vi "PH_Beckhoff-16BB.destructor.vi"(0 "i ref in":refnum<vi>, 5 "error in(no error)":errorcluster) -> (19 "error out":errorcluster)   [LabVIEW 2014, in "PH_Beckhoff-16BB.lvlib"]
doc: "This is the destructor of a class.\n\nLicense Agreement for this software:\n\nCopyright (C)\nGesellschaft für Schwerionenforschung, GSI\nPlanckstr. 1\n64291 Darmstadt\nGermany\n\nContact: D.Beck@gsi.de \n\nThis program is free software; you can redistribute it and/or modify it under the terms of the \nGNU General Public License as published by the Free Software Foundation; either version 2 of \nthe license, or (at your option) any later version.\n\nThis program is distributed in the hope that it will be useful, but WITHOUT ANY WARRANTY; \nwithout even the implied warranty of MERCHANTABILITY or FITNESS FOR A PARTICULAR PURPOSE. See the GNU General License for more details (http://www.gnu.org).\n\nGesellschaft für Schwerionenforschung, GSI\nPlanckstr. 1, 64291 Darmstadt, Germany\nFor all questions and ideas contact: M.Richter@gsi.de, H.Brand@gsi.de or D.Beck@gsi.de.\nLast update: 16-JUN-2004"
uses:
  PH_Beckhoff-16BB.lvlib
  PH_Beckhoff/PH_Beckhoff.lvlib
  CSlibraries-extern/DimLVEvent/LVDimInterface/LVDimInterface.lvlib
  CS_Core/CSSystem/CSSystemLib/CSSystemLib.lvlib
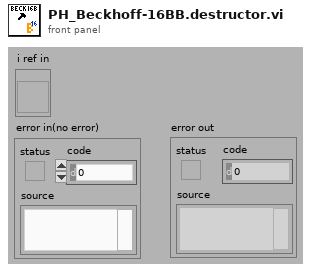
[diagram p1: front panel]
types:
  T1 = typedef "PH_Beckhoff-16BB.lvlib/PH_Beckhoff-16BB.i attribute.ctl" = cluster{"PA Chiller":cluster{"PSDB":cluster{"Status Service ID":i32, "Instance ID":i32, "Data Status":T2, "Ref Status":refnum<vi>, "Error Code":i32}, "Status":cluster{"GUI Ref":refnum<vi>, "Status Service ID":i32, "Status":T3}, "DIs":cluster{"Flow Control":cluster{"GUI Ref":refnum<vi>, "# in Data":i32}, "High-Temp":cluster{"GUI Ref":refnum<vi>, "# in Data":i32}, "Conductivity":cluster{"GUI Ref":refnum<vi>, "# in Data":i32}, "Niveau":cluster{"GUI Ref":refnum<vi>, "# in Data":i32}}, "PSDB Thread":cluster{"Ref":refnum<vi>, "Q-Ref":refnum<queue>}}, "PSDB":cluster{"Shot #":i32, "Subsystem":T4}, "Racktype":string, "PSDB Credentials":T5}
  T2 = typedef "PH_PSDBWriter.lvlib/PH_PSDBWriter.Data Status.ctl" = i16
  T3 = typedef "PH_StatusHandler.lvlib/PH_StatusHandler.Status.ctl" = i16
  T4 = typedef "PH_PSDBWriter.lvlib/PH_PSDBWriter.PHELIX-Subsystems.ctl" = i32
  T5 = typedef "PH_Common.lvlib/PH_Connection.PSDB Credentials.ctl" = cluster{"PW":string, "ID":string, "DS":string}
  T6 = enum16{"SetAttribute", "GetAttribute", "CreateAttribute", "DestroyAttribute", "DestroyAllAtributes"}
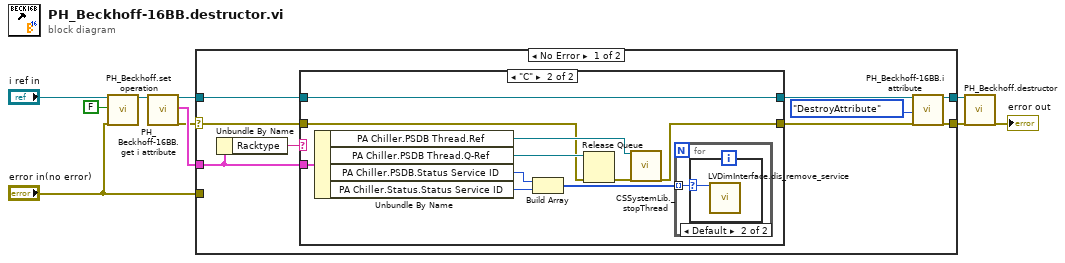
[diagram p0: block diagram]
diagram:
  n1 = call "PH_Beckhoff.set operation.vi"("VI in"="i ref in", "operation?"=FALSE, "error in (no error)"="error in(no error)") -> ("VI out"=w3:refnum<vi>)  [unwired: 15 in, 1 out]
  n2 = call "PH_Beckhoff-16BB.get i attribute.vi"("i ref in"=w3) -> ("i ref out"=w9:refnum<vi>, "i attribute"=w8:T1, "error out"=w7:errorcluster)  [unwired: 16 in]
  n3 = case shown="No Error" w7 {
    selector: w7 -> [w18 _]
    tunnel: [w14 w35] -> w6
    tunnel: [w13 w34] -> w10
    tunnel: "error in(no error)" -> [_ w34]
    tunnel: w9 -> [w19 w35]
    tunnel: w8 -> [w17 _]
    frame No Error {
      n4 = Unbundle By Name(w17) -> ("Racktype"=w16:string)
      n5 = case shown="\"C\"" w16 {
        tunnel: w19 -> [w21 w23]
        tunnel: w18 -> [w20 w24]
        tunnel: [w21 w23] -> w15
        tunnel: [w20 w22] -> w12
        tunnel: w17 -> [_ w31]
        frame Default {
        }
        frame "C" {
          n6 = Unbundle By Name(w31) -> ("PA Chiller.PSDB Thread.Ref"=w25:refnum<vi>, "PA Chiller.PSDB Thread.Q-Ref"=w26:refnum<queue>, "PA Chiller.PSDB.Status Service ID"=w30:i32, "PA Chiller.Status.Status Service ID"=w28:i32)
          n7 = Build Array(w30, w28) -> (w29:i32[])
          n8 = Release Queue(queue=w26, error in (no error)=w24) -> (error out=w27:errorcluster)  [unwired: 1 in, 2 out]
          n9 = call "CSSystemLib._stopThread.vi"("i ref in"=w25, "error in (no error)"=w27) -> ("error out"=w22:errorcluster)  [unwired: 16 in, 1 out]
          n10 = for {
            tunnel: w29 -> [w32] mode=indexing
            n11 = case shown="Default" w32 {
              selector: w32 -> [_ w33]
              frame -1 {
              }
              frame Default {
                n12 = call "LVDimInterface.dis_remove_service.vi"("my_serviceID"=w33) -> ()  [unwired: 18 in, 1 out]
              }
            }
          }
        }
      }
      n13 = call "PH_Beckhoff-16BB.i attribute.vi"("VI Refnum"=w15, "Action"=T6."DestroyAttribute", "error in (no error)"=w12) -> ("VI Refnum out"=w14:refnum<vi>, "error out"=w13:errorcluster)  [unwired: 14 in, 1 out]
    }
    frame Error {
    }
  }
  n14 = call "PH_Beckhoff.destructor.vi"("i ref in"=w6, "error in(no error)"=w10) -> ("error out"=→"error out":errorcluster)  [unwired: 17 in]
